vi "filter_interlock.vi"(6 "timeout (25000ms)":i32=25000, 8 "error in (no error)":errorcluster, 10 "check batch?":bool, 11 "daemon reference in":refnum<k5>) -> (0 "error out":errorcluster, 1 "present":bool, 2 "response":string, 3 "daemon reference out":refnum<k5>, 5 "command out":string="random")   [LabVIEW 2017]
doc: "<b>Command: </b>\"filter_interlock\"\n\n<b>Description: </b> This command return filter interlock status, 1 = filter present, 0= absence.\n\n<b>Parameters: </b> None\n____________________________________________\nDIPC 692 Daemon API 10.0.0.1\nSam Tee - Dyson Technology Ltd\nCopyright (c) 2024, Dyson Technology Ltd"
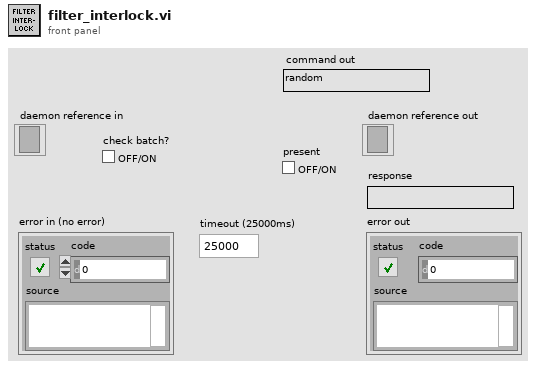
[diagram p1: front panel]
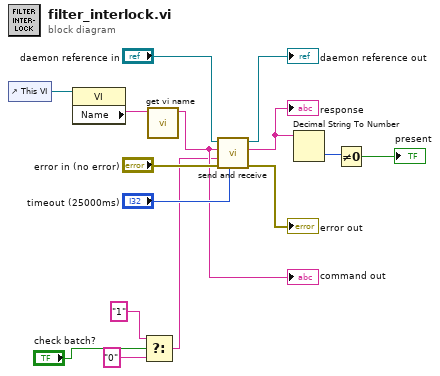
[diagram p0: block diagram]
diagram:
  n1 = control-ref of="This VI"() -> (w10:refnum<vi>)
  n2 = property class="VI"(reference=w10) -> ("Name"=w9:string)  [unwired: 1 in, 2 out]
  n3 = Select(t="1", s="check batch?", f="0") -> (s? t:f=w1:string)
  n4 = call "get vi name.vi"("library.lvlib:name.vi"=w9) -> ("vi name"=w8:string)  [unwired: 10 in]
  "command out" <- w8
  n5 = call "send and receive.vi"("timeout (25000ms)"="timeout (25000ms)", "error in (no error)"="error in (no error)", "data"=w1, "command"=w8, "daemon reference in"="daemon reference in") -> ("error out"=→"error out":errorcluster, "response"=w7:string, "daemon reference out"=→"daemon reference out":refnum<k5>)  [unwired: 4 in]
  "response" <- w7
  n6 = Decimal String To Number(string=w7) -> (number=w6:i32)  [unwired: 2 in, 1 out]
  n7 = Not Equal To 0?(x=w6) -> (x != 0?=→"present":bool)
